vi "Set Pause.vi"(8 "error in (no error)":errorcluster, 10 "Pause":bool, 11 "FormulaG API in":refnum<class "FormulaG API.lvclass">) -> (0 "error out":errorcluster, 3 "FormulaG API out":refnum<class "FormulaG API.lvclass">)   [LabVIEW 2024, in "FormulaG.lvlib" / "FormulaG API.lvclass"]
uses:
  FormulaG API.lvclass
  Command.ctl
  FormulaG API.lvclass/FormulaG API.ctl
  <vilib>/IlluminatedG/IG GodotServer/GodotLV/GodotServer/GodotServer.lvclass
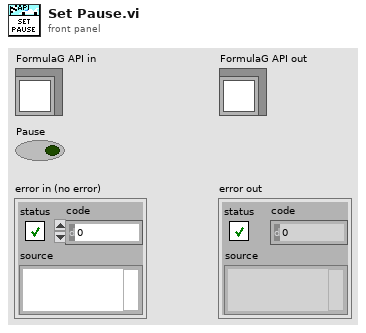
[diagram p1: front panel]
types:
  T1 = enum16{"big-endian, network order", "native, host order", "little-endian"}
  T2 = typedef "FormulaG.lvlib/FormulaG API.lvclass/Command.ctl" = enum8{"None", "Reset Car", "Request State", "Control Car", "Request Info", "Set Options", "Set Camera", "Set Pause", "Request Time"}
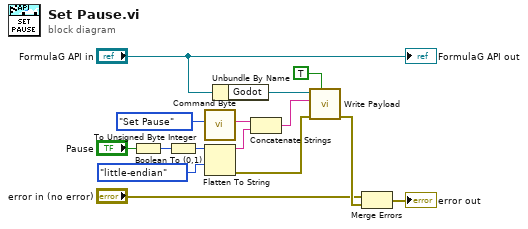
[diagram p0: block diagram]
diagram:
  n1 = Boolean To (0,1)(Boolean="Pause") -> (0, 1=w6:i16)
  n2 = To Unsigned Byte Integer(number=w6) -> (unsigned 8bit integer=w5:u8)
  n3 = call "Command Byte.vi"("Command"=Command."Set Pause") -> ("Command Byte"=w14:string)  [unwired: 10 in]
  n4 = Flatten To String(anything=w5, byte order (0:big-endian, network order)=T1."little-endian") -> (data string=w10:string, error out=w9:errorcluster)  [unwired: 2 in, 1 out]
  n5 = Unbundle By Name("FormulaG API in") -> ("Godot"=w13:refnum<class "GodotServer.lvclass">)
  n6 = Concatenate Strings(w14, w10) -> (w12:string)
  n7 = call <vilib>:"Write Payload.vi"("Binary (F = Text)"=TRUE, "error in (no error)"=w9, "Payload"=w12, "GodotServer in"=w13) -> ("error out"=w8:errorcluster)  [unwired: 6 in, 1 out]
  n8 = Merge Errors("error in (no error)", w8) -> (→"error out":errorcluster)
  "FormulaG API out" <- "FormulaG API in"
